vi "Ranged_Duty_Cycle.vi"(8 "Volt Input":dbl) -> (3 "Duty Cycle":dbl)   [LabVIEW 2016]
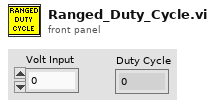
[diagram p1: front panel]
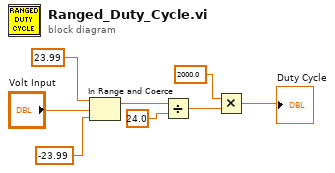
[diagram p0: block diagram]
diagram:
  n1 = In Range and Coerce(upper limit=23.99, x="Volt Input", lower limit=-23.99) -> (coerced(x)=w5:dbl)  [unwired: 1 out]
  n2 = Divide(x=w5, y=24.0) -> (x/y=w3:dbl)
  n3 = Multiply(x=2000.0, y=w3) -> (x*y=→"Duty Cycle":dbl)
